vi "ziExample-Boxcar.vi"() -> ()   [LabVIEW 2009]
doc: "Control a Zurich instrument device via the LabOne Labview API. \nRequirements: Zurich Instruments UHFLI \nThis example retrives boxcar samples from a Zurich Instruments UHFLI instrument.\n\n© Zurich Instruments AG, www.zhinst.com"
uses:
  <instrlib>/Zurich Instruments LabOne/Public/Configure/ziSetValueDoubleArray.vi
  <instrlib>/Zurich Instruments LabOne/Public/Utility/ziTicksToS_vector.vi
  <instrlib>/Zurich Instruments LabOne/Public/Data/ziGetEventDoubleDataTS.vi
  <instrlib>/Zurich Instruments LabOne/Public/Utility/ziTicksToS_single.vi
  <instrlib>/Zurich Instruments LabOne/Zurich Instruments LabOne.lvlib
panel:
  out "Error Out":errorcluster
  out "Sample Rate (1/s)":cluster{"Timestamp(s)":dbl[], "Value":dbl[]}(graph)
  in  "Address":string="DEV"
  out "Selected Device":string
  out "Update Rate (1/s)":dbl(graph)
  out "All Values (V)":cluster{"Timestamp(s)":dbl[], "Value":dbl[]}(graph)
  out "Single Values":dbl format="%#_6p"
  in  "stop":bool
  # "ziExample-Boxcar.vi\nRequirements: UHFLI\nsee block diagram for VI description"
  # "Tested Devices:\n- UHFLI"
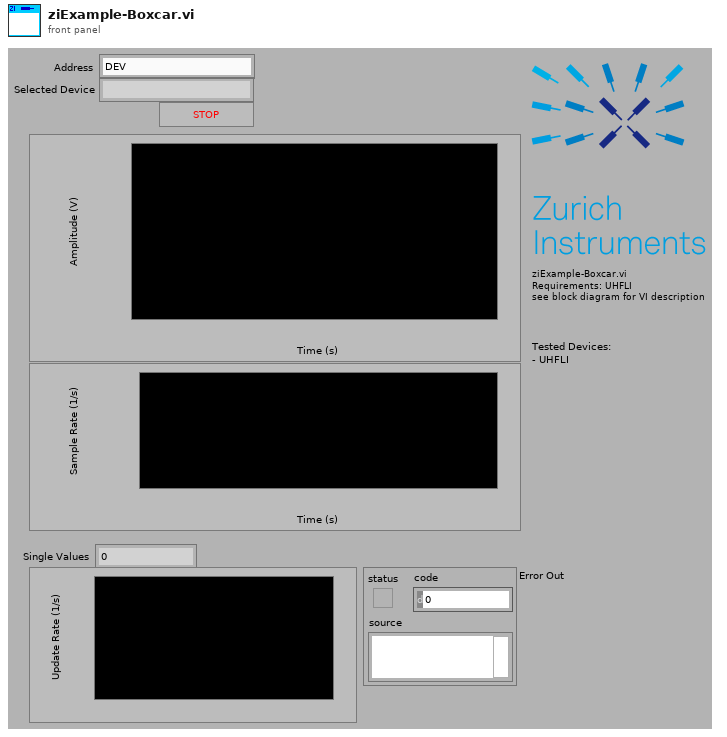
[diagram p1: front panel]
types:
  T1 = typedef "Zurich Instruments LabOne.lvlib/ziTypeHandle.ctl" = cluster{"handleValid":bool, "Conn":u64, "Path Prefix":string, "Handle":u64, "Connected":bool, "Clockbase(s)":dbl}
  T2 = typedef "Zurich Instruments LabOne.lvlib/ziTypeDoubleDataTS.ctl" = cluster{"Timestamp (ticks)":u64[], "Value":dbl[]}
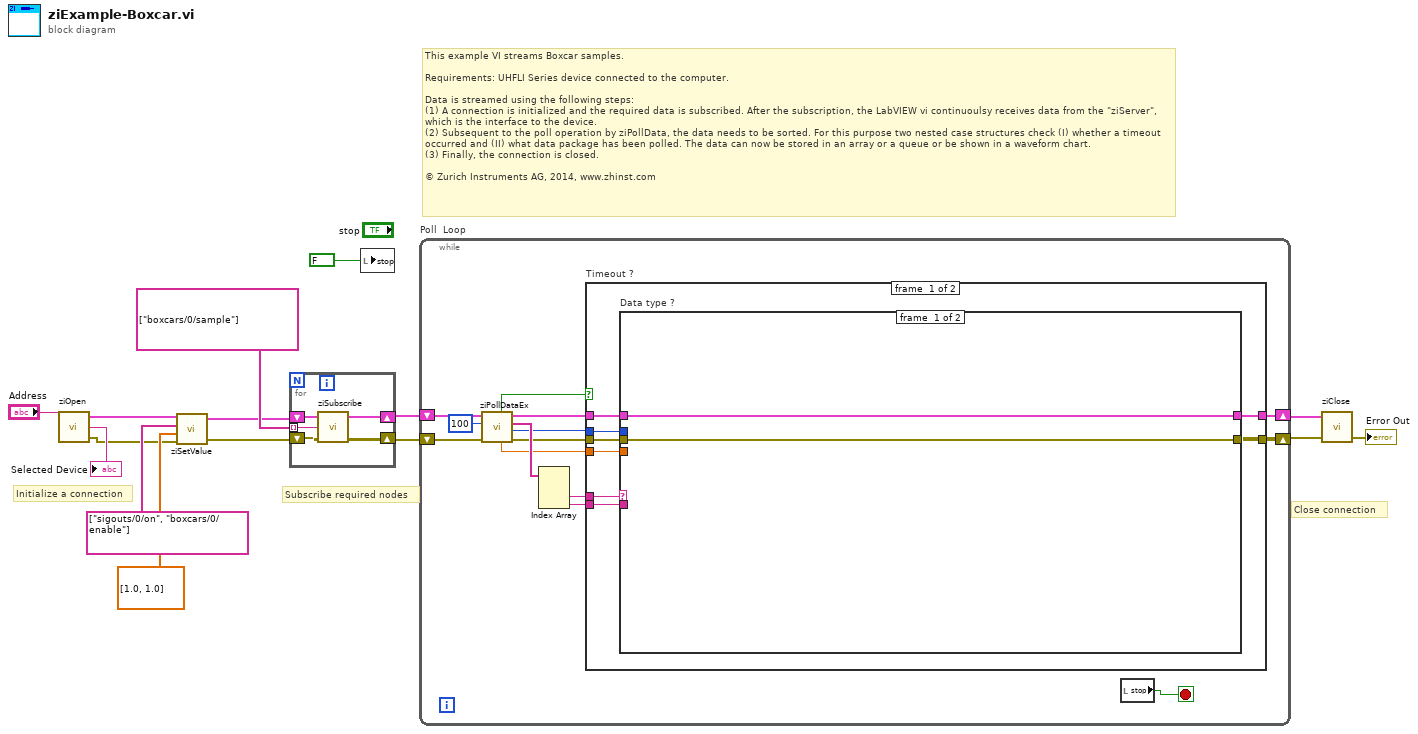
[diagram p0: block diagram]
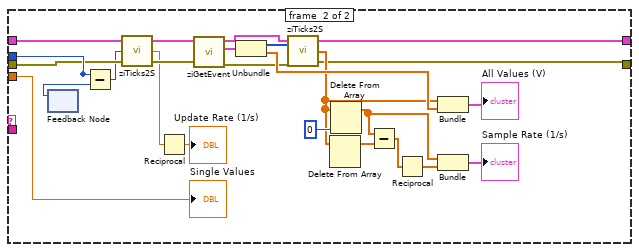
[diagram p2: hidden frame]
diagram:
  # "Close connection"
  # "Initialize a connection"
  # "Subscribe required nodes"
  # "This example VI streams Boxcar samples.\n\nRequirements: UHFLI Series device connected to the computer.\n\nData is streamed using the following steps:\n(1) A connection is initialized and the required data is subscribed. After the subscription, the LabVIEW vi continuoulsy receives data from the \"ziServer\", which is the interface to the device. \n(2) Subsequent to the poll operation by ziPollData, the data needs to be sorted. For this purpose two nested case structures check (I) whether a timeout occurred and (II) what data package has been polled. The data can now be stored in an array or a queue or be shown in a waveform chart. \n(3) Finally, the connection is closed. \n\n© Zurich Instruments AG, 2014, www.zhinst.com"
  n1 = call <instrlib>:"ziOpen.vi"("Address"="Address") -> ("Error Out"=w4:errorcluster, "Selected Device"=→"Selected Device":string, "HandleOut"=w5:T1)  [unwired: 1 in, 2 out]
  n2 = call-poly <instrlib>:"ziSetValue.vi"("Error In"=w4, "Values"=dbl[] [1.0, 1.0], "Paths"=string[] ["sigouts/0/on", "boxcars/0/enable"], "Handle In"=w5) -> ("Error Out"=w3:errorcluster, "Handle Out"=w2:T1)  [unwired: 1 in]
  n3 = for {
    shift-right: [w20] -> w11
    shift-left: w2 -> [w18]
    shift-right: [w19] -> w10
    shift-left: w3 -> [w17]
    tunnel: string[] ["boxcars/0/sample"] -> [w16] mode=indexing
    n4 = call <instrlib>:"ziSubscribe.vi"("error in"=w17, "Path ()"=w16, "Handle In"=w18) -> ("error out"=w19:errorcluster, "Handle Out"=w20:T1)  [unwired: 1 in]
  }
  n5 = local write "stop"(FALSE ("Record")) -> ()
  n6 = while "Poll  Loop" {
    shift-right: [w25] -> w12
    shift-left: w11 -> [w34]
    shift-right: [w23] -> w13
    shift-left: w10 -> [w33]
    stop <- w31 stop-if-true
    n7 = call <instrlib>:"ziPollDataEx.vi"("error in"=w33, "Timeout ms (50)"=100 ("TimeOut ms (50)"), "Handle In"=w34) -> ("error out"=w24:errorcluster, "Timestamp (ticks)"=w27:u64, "PathArray"=w29:string[], "Handle Out"=w26:T1, "Value Double"=w22:dbl, "Timed Out"=w30:bool)  [unwired: 1 in, 2 out]
    n8 = Index Array(array=w29) -> (element #2=w28:string, element #3=w21:string)  [unwired: 3 in, 1 out]
    n9 = case "Timeout ?" shown="False" w30 {
      tunnel: w28 -> [w42 _]
      tunnel: w27 -> [w41 _]
      tunnel: w26 -> [w40 w71]
      tunnel: [w39 w71] -> w25
      tunnel: w24 -> [w38 w70]
      tunnel: [w37 w70] -> w23
      tunnel: w22 -> [w36 _]
      tunnel: w21 -> [w35 _]
      frame #0 {
        n10 = case "Data type ?" shown="\"BOXCARS\"" w42 {
          tunnel: w41 -> [_ w68]
          tunnel: w40 -> [w44 w67]
          tunnel: [w44 w49] -> w39
          tunnel: w38 -> [w43 w66]
          tunnel: [w43 w46] -> w37
          tunnel: w36 -> [_ w69]
          tunnel: w35 -> [_ _]
          frame #0 {
          }
          frame #1 {
            n11 = feedback #1() -> (w63:u64)  [unwired: 1 in]
            n12 = Subtract(x=w68, y=w63) -> (x-y=w62:u64)
            n13 = call-poly <instrlib>:"ziTicks2S.vi"("Error In"=w66, "Timestamp(ticks)"=w62, "Handle In"=w67) -> ("Error Out"=w60:errorcluster, "Timestamp(s)"=w59:dbl, "Handle Out"=w61:T1)
            n14 = Reciprocal(x=w59) -> (1/x=→"Update Rate (1/s)":dbl)
            n15 = call-poly <instrlib>:"ziGetEvent.vi"("Error In"=w60, "Handle In"=w61) -> ("Error Out"=w48:errorcluster, "Sample Out"=w65:T2, "Handle Out"=w47:T1)  [unwired: 7 in]
            n16 = Unbundle(w65) -> ("Timestamp (ticks)"=w52:u64[], "Value"=w53:dbl[])
            n17 = call-poly <instrlib>:"ziTicks2S.vi"("Error In"=w48, "Timestamp (ticks)"=w52, "Handle In"=w47) -> ("Error Out"=w46:errorcluster, "Timestamp(s)"=w50:dbl[], "Handle Out"=w49:T1)
            n18 = Delete From Array(array=w50) -> (array with subset deleted=w58:dbl[])  [unwired: 2 in, 1 out]
            n19 = Delete From Array(array=w50, index=0) -> (array with subset deleted=w45:dbl[])  [unwired: 1 in, 1 out]
            n20 = Subtract(x=w45, y=w58) -> (x-y=w51:dbl[])
            n21 = Reciprocal(x=w51) -> (1/x=w55:dbl[])
            n22 = Bundle("Timestamp(s)"=w50, "Value"=w53) -> (→"All Values (V)":cluster{"Timestamp(s)":dbl[], "Value":dbl[]})  [unwired: 1 in]
            n23 = Bundle("Timestamp(s)"=w45, w55) -> (→"Sample Rate (1/s)":cluster{"Timestamp(s)":dbl[], dbl[]})  [unwired: 1 in]
            "Single Values" <- w69
          }
        }
      }
      frame #1 {
        # "Timeout, no action."
      }
    }
    n24 = local read "stop"() -> (w31:bool)
  }
  n25 = call <instrlib>:"ziClose.vi"("Error In"=w13, "Handle In"=w12) -> ("Error Out"=→"Error Out":errorcluster)  [unwired: 3 out]
